vi "题目3.vi"() -> ()   [LabVIEW 2017]
uses:
  <vilib>/measure/NI_MABase.lvlib
panel:
  out "Y":dbl[](array[numeric])
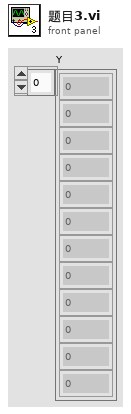
[diagram p1: front panel]
types:
  T1 = enum16{"open", "replace", "create", "open or create", "replace or create", "replace or create with confirmation"}
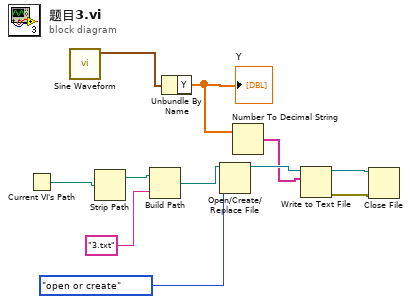
[diagram p0: block diagram]
diagram:
  n1 = Current VI's Path() -> (path=w10:path)
  n2 = call <vilib>:"Sine Waveform.vi"() -> ("signal out"=w11:waveform(dbl))  [unwired: 10 in, 1 out]
  n3 = Strip Path(path=w10) -> (stripped path=w9:path)  [unwired: 1 out]
  n4 = Build Path(base path=w9, name or relative path="3.txt" ("名称或相对路径")) -> (appended path=w7:path)
  n5 = Unbundle By Name(w11) -> ("Y"=w4:dbl[])
  "Y" <- w4
  n6 = Open/Create/Replace File(file path (use dialog)=w7, operation (0:open)=T1."open or create" ("操作(0:open)")) -> (refnum out=w5:refnum<file>)  [unwired: 4 in, 2 out]
  n7 = Number To Decimal String(number=w4) -> (decimal integer string=w3:string[])  [unwired: 1 in]
  n8 = Write to Text File(file (use dialog)=w5, text=w3) -> (refnum out=w2:refnum<file>, error out=w1:errorcluster)  [unwired: 2 in, 1 out]
  n9 = Close File(refnum=w2, error in=w1) -> ()  [unwired: 2 out]
